vi "Unit Test.vi"() -> ()   [LabVIEW 2019, in "sbRIO9623.lvlib"]
uses:
  sbRIO9623.lvlib
  User Event/Controls/UE Abort Action.ctl
panel:
  in  "Close":bool
  in  "Open":bool
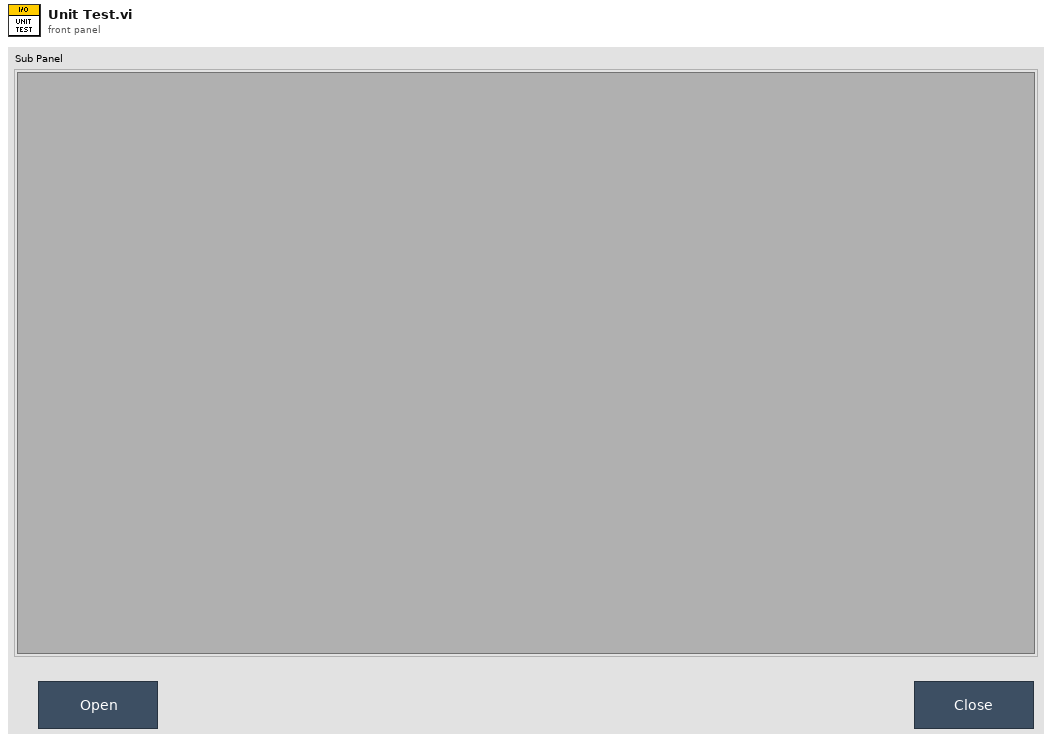
[diagram p1: front panel]
types:
  T1 = typedef "UE Abort Action.ctl" = enum16{"Create", "Get", "Destroy"}
  T2 = typedef "sbRIO9623.lvlib/SEQ Data.ctl" = cluster{"Lid Sensor 1":bool, "Lid Sensor 2":bool, "Laser Interlock":bool, "Buffer Tank":bool, "Wash Tank":bool, "Waste Tank":bool, "SiPM 1":fxp<+,20,5>, "SiPM 2":fxp<+,20,5>, "Initialize Success?":bool, "VI Refnum":refnum<vi>}
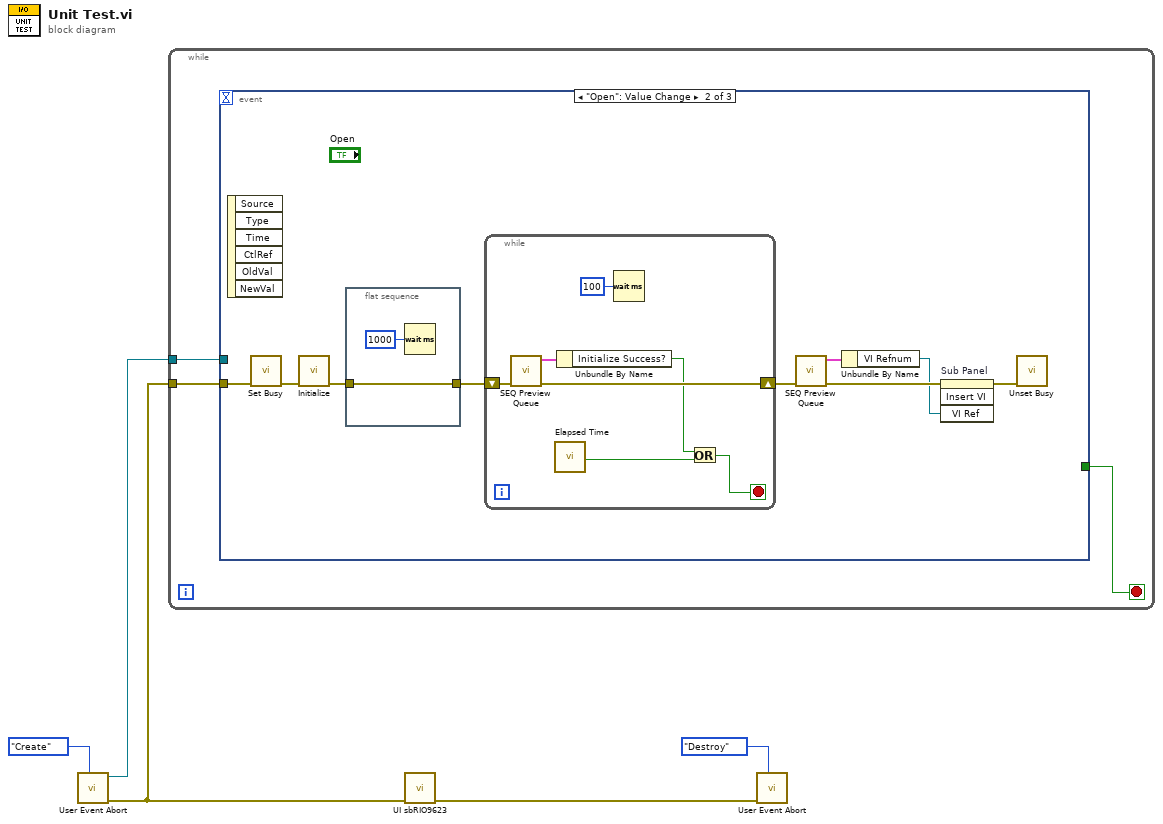
[diagram p0: block diagram]
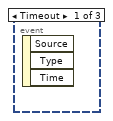
[diagram p2: hidden frame]
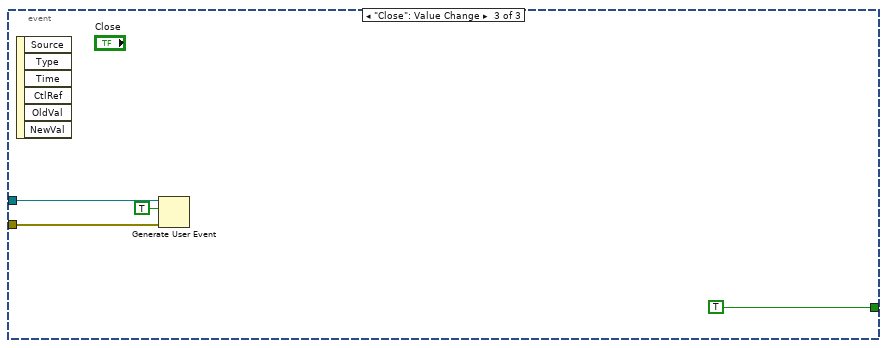
[diagram p3: hidden frame]
diagram:
  n1 = call "User Event Abort.vi"("Action"=UE_Abort_Action."Create") -> ("Error Out"=w1:errorcluster, "User Event Out"=w2:refnum<user-event>)  [unwired: 9 in]
  n2 = while {
    tunnel: w2 -> [w8]
    tunnel: w1 -> [w7]
    stop <- w6 stop-if-true
    n3 = event shown="[1] \"Open\": Value Change" {
      selector: _ -> [_ _ _]
      dyn-events: _ -> [_ _ _]
      timeout: _ -> [_ _ _]
      tunnel: w8 -> [_ _ w30]
      tunnel: w7 -> [_ w17 w29]
      tunnel: [_ _ TRUE] -> w6
      event Timeout {
        n4 = event-data() -> ()  [unwired: 1 in, 3 out]
      }
      event "Open": Value Change {
        n5 = event-data() -> ()  [unwired: 1 in, 6 out]
        n6 = call <vilib>:"Set Busy.vi"("error in (no error)"=w17) -> ("error out"=w16:errorcluster)  [unwired: 9 in, 1 out]
        n7 = call "Initialize.vi"("Error In"=w16) -> ("Error Out"=w15:errorcluster)  [unwired: 10 in]
        n8 = flat-sequence {
          tunnel: w15 -> [w25]
          tunnel: [w25] -> w14
          frame #0 {
            n9 = Wait (ms)(milliseconds to wait=u32 1000) -> ()  [unwired: 1 out]
          }
        }
        n10 = while {
          shift-right: [w23] -> w13
          shift-left: w14 -> [w24]
          stop <- w20 stop-if-true
          n11 = call "SEQ Preview Queue.vi"("error in"=w24) -> ("error out"=w23:errorcluster, "SEQ Data"=w22:T2)  [unwired: 9 in]
          n12 = call "Elapsed Time"() -> ("Time has Elapsed"=w19:bool)  [unwired: 12 in, 7 out]
          n13 = Unbundle By Name(w22) -> ("Initialize Success?"=w21:bool)
          n14 = Wait (ms)(milliseconds to wait=u32 100) -> ()  [unwired: 1 out]
          n15 = Or(x=w21, y=w19) -> (x .or. y?=w20:bool)
        }
        n16 = call "SEQ Preview Queue.vi"("error in"=w13) -> ("error out"=w11:errorcluster, "SEQ Data"=w12:T2)  [unwired: 9 in]
        n17 = Unbundle By Name(w12) -> ("VI Refnum"=w9:refnum<vi>)
        n18 = invoke on="Sub Panel" class="SubPnl" method="Insert VI"(error in=w11, "VI Ref"=w9) -> (error out=w10:errorcluster)  [unwired: 2 in, 3 out]
        n19 = call <vilib>:"Unset Busy.vi"("error in (no error)"=w10) -> ()  [unwired: 10 in, 1 out]
      }
      event "Close": Value Change {
        n20 = event-data() -> ()  [unwired: 1 in, 6 out]
        n21 = Generate User Event(user event=w30, event data cluster=TRUE ("event data"), error in=w29) -> ()  [unwired: 1 in, 2 out]
      }
    }
  }
  n22 = call "UI sbRIO9623.vi"("error in"=w1) -> ("error out"=w5:errorcluster)  [unwired: 10 in]
  n23 = call "User Event Abort.vi"("Action"=UE_Abort_Action."Destroy", "Error In"=w5) -> ()  [unwired: 8 in, 2 out]
